vi "End Sync Box.vi"(8 "error in (no error)":errorcluster, 11 "Channel in":refnum<class "Channel.lvclass">) -> (0 "error out":errorcluster, 3 "Channel out":refnum<class "Channel.lvclass">)   [LabVIEW 2018, in "Channel.lvclass"]
uses:
  Channel.lvclass
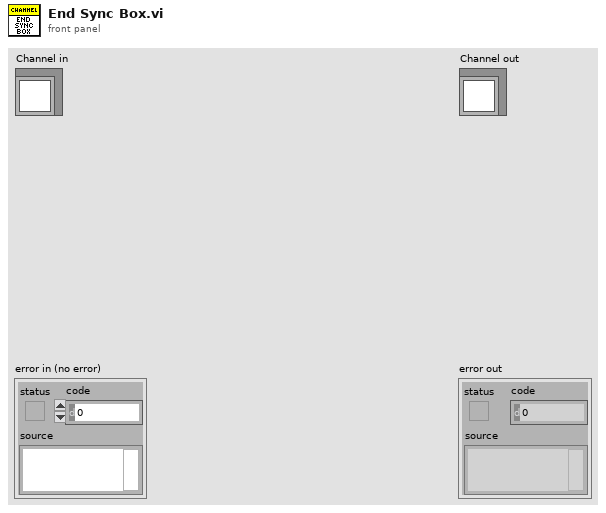
[diagram p1: front panel]
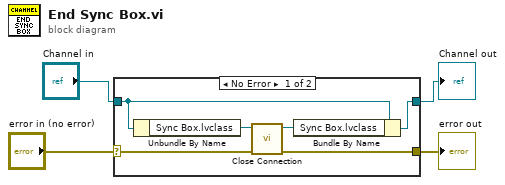
[diagram p0: block diagram]
diagram:
  n1 = case shown="No Error" "error in (no error)" {
    selector: "error in (no error)" -> [w9 w12]
    tunnel: [w10 w12] -> w3
    tunnel: [w5 w11] -> w1
    tunnel: "Channel in" -> [w6 w11]
    frame No Error {
      n2 = Unbundle By Name(w6) -> ("Sync Box.lvclass"=w8:refnum<class "Sync Box.lvclass">)
      n3 = call "Close Connection.vi"("error in (no error)"=w9, "Sync Box in"=w8) -> ("error out"=w10:errorcluster, "Sync Box out"=w7:refnum<class "Sync Box.lvclass">)  [unwired: 8 in]
      n4 = Bundle By Name(cluster=w6, "Sync Box.lvclass"=w7) -> (w5:refnum<class "Channel.lvclass">)
    }
    frame Error {
    }
  }
  "error out" <- w3
  "Channel out" <- w1
